vi "Destructor.vi"(8 "error in":errorcluster, 11 "FailureReference in":refnum<class "FailureReference.lvclass">) -> (0 "error out":errorcluster)   [LabVIEW 2021, in "ProligentXMLGenerator.lvlib" / "FailureReference.lvclass"]
uses:
  FailureReference.lvclass
  FailureReference.lvclass/FailureReference.ctl
  Model/CustomData/CustomData.lvclass
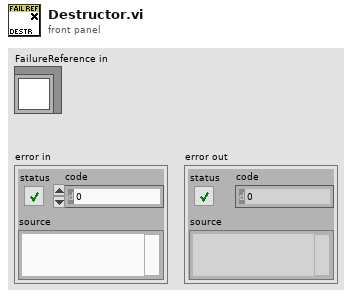
[diagram p1: front panel]
types:
  T1 = typedef "ProligentXMLGenerator.lvlib/FailureReference.lvclass/Data.ctl" = cluster{"Name":string, "CustomData":refnum<class "CustomData.lvclass">, "Id":refnum<class "Guid.lvclass">}
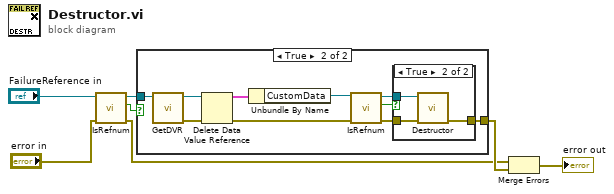
[diagram p0: block diagram]
diagram:
  n1 = call "IsRefnum.vi"("error in"="error in", "FailureReference in"="FailureReference in") -> ("error out"=w1:errorcluster, "IsRefnum"=w3:bool, "FailureReference out"=w4:refnum<class "FailureReference.lvclass">)  [unwired: 7 in]
  n2 = case shown="True" w3 {
    tunnel: [_ w11] -> w5
    tunnel: w4 -> [_ w8]
    frame False {
    }
    frame True {
      n3 = call "GetDVR.vi"("FailureReference in"=w8) -> ("error out"=w16:errorcluster, "DVRReference"=w17:refnum<data-value>)  [unwired: 9 in]
      n4 = Delete Data Value Reference(data value reference=w17, error in=w16) -> (data value=w15:T1, error out=w9:errorcluster)
      n5 = Unbundle By Name(w15) -> ("CustomData"=w12:refnum<class "CustomData.lvclass">)
      n6 = call "IsRefnum.vi"("error in"=w9, "CustomDataType in"=w12) -> ("error out"=w14:errorcluster, "IsRefnum"=w13:bool, "CustomDataType out"=w10:refnum<class "CustomData.lvclass">)  [unwired: 7 in]
      n7 = case shown="True" w13 {
        tunnel: w14 -> [w18 w21]
        tunnel: [w18 w20] -> w11
        tunnel: w10 -> [_ w19]
        frame False {
        }
        frame True {
          n8 = call "Destructor.vi"("error in"=w21, "CustomDataType"=w19) -> ("error out"=w20:errorcluster)  [unwired: 9 in]
        }
      }
    }
  }
  n9 = Merge Errors(w1, w5) -> (→"error out":errorcluster)
